vi "UHR-Fleezers Control (host) -Leonardo 04-2018 V3.vi"(0 "Tab Control":T5(tab)=enum."Trap Control (RF)") -> ()   [LabVIEW 2013] (continued)
  n81 = local write "Update Count (MCL)"(w134) -> ()
  n82 = local write "Total Counts (ticks)"(w134) -> ()
  n83 = local write "Ave. Period (s)"(w200) -> ()
  n84 = property on="2D or 1D Scan" class="Bool (strict)"("Val(Sgnl)"=w154) -> ()  [unwired: 2 in, 2 out]
  n85 = xnode "Read/Write Control"("FPGA VI Reference In"=w151, "error in"=w171, "ai count"="AI Count (ticks)", "Interlace ON/OFF"=w137, "Number Interlace Cycles"=w136, "Set 1"=w14, "Set 2"=w13, "Set 3"=w12, "FB On/Off Set 1"=w258, "FB On/Off Set 2"=w257, "Interlace Off Parameters"=w135, "FB Setpoint Set 1"=w249, "FB Setpoint Set 2"=w248, "FB Gains"="PID gains", "FB output range"=cluster{"output high":i16, "output low":i16} {"output high"=3000, "output low"=0} ("FB output range 1"), "Cycles per step"=w234, "Scan BD"=w246, "Number of scans"=w230, "Scan steps"=w235, "Scan freq.  increment"=w236, "AO1 (Y)"=w218, "AO2 (X)"=w217, "Scan freq.  increment (MCL)"=w211, "Scan steps (MCL)"=w210, "Cycles per step (MCL)"=w209, "Number of scans (MCL)"=w208, "MCL count"=w134, "Cont. Scan (MCL)"=w207, "MCL Scan Axis"=w201, "1D or 2D Scan?"=w154, "N of AI1 Int Acq Sets"=w191, "BD 1 Delay (ticks)"="Freq switch delay", "Amp switch delay"="Amp switch delay", "Swap F1 and F2"="Swap F1 and F2", "APD Acq Rate Count"=w159, "APD to FIFO"=FALSE, "APD Gate Operating Mode"="APD Gate", "APD Gate ON Count"="APD Gate ON Count", "APD Gate OFF Count"="APD Gate OFF Count", "Invert APD Gate"="Invert APD Gate", "DIO count 1 (ticks)"="DIO count 1 (ticks)", "DIO count 2 (ticks)"="DIO count 2 (ticks)", "DIO count 3 (ticks)"="DIO count 3 (ticks)", "APD 1 AO scale factor"="APD 1 AO Mult.", "APD 2 AO scale factor"="APD 2 AO Mult.", "Diff FB Measurement?"=w19, "Dynamic Force FB (Ronen)"=w18, "Negate Diff?"=w17, "Next trap write delay (ticks)"="Next trap write delay (ticks)", "Phase offset method"="Phase offset method", "Phase Trap 1"="Phase increment trap 1", "RF phase reset before cycles"="RF phase reset before cycles", "Phase Trap 2"="Phase increment trap 2") -> ("FPGA VI Reference Out"=w129:T20, "error out"=w131:errorcluster)  [unwired: 1 in]
  n86 = local read "Green Laser ON/Interlacing"() -> (w132:bool)
  n87 = local read "Green laser mode"() -> (w133:enum32{"Laser ON", "Laser OFF", "Interlace"})
  n88 = local read "GI Frequency, OFF count"() -> (w125:u32)
  n89 = local read "GI Frequency, ON count"() -> (w124:u32)
  n90 = Multiply(x="Current When FB OFF (%)", y=655.35) -> (x*y=w115:dbl)
  n91 = local read "Green FB Count"() -> (w123:u32)
  n92 = Multiply(x="Green FB Setpoint (mV)", y=3.2767) -> (x*y=w112:dbl)
  n93 = To Unsigned Word Integer(number=w115) -> (unsigned 16bit integer=w113:u16)
  n94 = local read "Invert GI"() -> (w127:bool)
  n95 = To Word Integer(number=w112) -> (16bit integer=w110:i16)
  n96 = case shown="True" w132 {
    tunnel: w133 -> [_ w293]
    tunnel: [enum32{"Laser ON", "Laser OFF", "Interlace"}."Laser OFF" ("Green laser mode") w293] -> w126
    frame False {
    }
    frame True {
    }
  }
  n97 = local read "Trap Pos. AI1 X Pre-scale"() -> (w81:u16)
  n98 = local read "Trap Pos FB Monitor\nT1 or T2"() -> (w88:bool)
  n99 = local read "Trap Pos FB Int Count"() -> (w76:u16)
  n100 = local read "Trap Pos FB Negate Action"() -> (w87:bool)
  n101 = local read "Trap Pos. FB Offset Factor"() -> (w86:i64)
  n102 = local read "Trap Pos. FB Mult Factor"() -> (w85:i64)
  n103 = local read "Trap Pos. FB Gains"() -> (w83:T11)
  n104 = local read "Trap Pos. FB Range"() -> (w84:T12)
  n105 = xnode "Read/Write Control"("FPGA VI Reference In"=w129, "error in"=w131, "Green interlace ON count 2"=w124, "Green interlace OFF count 2"=w125, "Invert GI 2"=w127, "Operating Mode 2"=w126, "Green FB Gains"="Green FB Gains", "Green FB Setpoint"=w110, "Green FB On/Off"="Green FB On/Off", "Current Out"=w113, "Green int current ON count adj"="Green int current ON count adj", "Green FB Count"=w123, "Operating Mode"=w126, "Green interlace OFF count"=w125, "Green interlace ON count"=w124, "Invert GI"=w127, "Trap Pos FB Monitor T1 or T2"=w88, "Trap Pos FB Negate Action"=w87, "Trap Pos. FB Offset Factor"=w86, "Trap Pos. FB Mult Factor"=w85, "Trap pos. FB Range"=w84, "Trap Pos. FB Gains"=w83, "Force feedback"=FALSE, "AI1 X Scale"=w81, "Trap Pos to FIFO"=TRUE, "Trap Pos FB Int Count"=w76) -> ("FPGA VI Reference Out"=w128:T20, "error out"=w130:errorcluster)
  n106 = xnode "Invoke Method"("FPGA VI Reference In"=w128, "error in"=w130, "Requested Depth"="Trap AI FIFO Depth") -> ("FPGA VI Reference Out"=w91:T20, "error out"=w90:errorcluster)  [unwired: 1 out]
  n107 = xnode "Invoke Method"("FPGA VI Reference In"=w91, "error in"=w90, "Requested Depth"="Trap Position FIFO Depth") -> ("FPGA VI Reference Out"=w78:T20, "error out"=w77:errorcluster)  [unwired: 1 out]
  n108 = flat-sequence {
    tunnel: w152 -> [w298]
    tunnel: [w298] -> w151
    tunnel: [w297] -> w35
    tunnel: [w296] -> w150
    tunnel: [w294] -> w148
    tunnel: [w295] -> w149
    frame #0 {
      w295 = T16 {"Minimum"=60.0, "Maximum"=90.0, "Increment"=1.0} ("Min Max Inc")
      w294 = T16 {"Minimum"=0.0, "Maximum"=75.0, "Increment"=1.0} ("Data Entry Limits")
      w297 = T16 {"Minimum"=60.0, "Maximum"=90.0, "Increment"=1.0} ("Min Max Inc")
      w296 = T16 {"Minimum"=0.0, "Maximum"=75.0, "Increment"=1.0} ("Data Entry Limits")
      n109 = property on="BD 2 Frequency 1 (MHz)" class="DigNum (strict)"("Data Range"=w295) -> ()  [unwired: 2 in, 2 out]
      n110 = property on="BD 2 Frequency 3 (MHz)" class="DigNum (strict)"("Data Range"=w295) -> ()  [unwired: 2 in, 2 out]
      n111 = property on="BD 2 Frequency 2 (MHz)" class="DigNum (strict)"("Data Range"=w295) -> ()  [unwired: 2 in, 2 out]
      n112 = property on="BD 1 Frequency 1 (MHz)" class="DigNum (strict)"("Data Range"=w297) -> ()  [unwired: 2 in, 2 out]
      n113 = property on="BD 1 Frequency 2 (MHz)" class="DigNum (strict)"("Data Range"=w297) -> ()  [unwired: 2 in, 2 out]
      n114 = property on="BD 1 Frequency 3 (MHz)" class="DigNum (strict)"("Data Range"=w297) -> ()  [unwired: 2 in, 2 out]
      n115 = property on="BD 2 Amplitude 1 (%)" class="DigNum (strict)"("Data Range"=w294) -> ()  [unwired: 2 in, 2 out]
      n116 = property on="BD 2 Amplitude 2 (%)" class="DigNum (strict)"("Data Range"=w294) -> ()  [unwired: 2 in, 2 out]
      n117 = property on="BD 2 Amplitude 3 (%)" class="DigNum (strict)"("Data Range"=w294) -> ()  [unwired: 2 in, 2 out]
      n118 = property on="BD 1 Amplitude 3 (%)" class="DigNum (strict)"("Data Range"=w296) -> ()  [unwired: 2 in, 2 out]
      n119 = property on="BD 1 Amplitude 2 (%)" class="DigNum (strict)"("Data Range"=w296) -> ()  [unwired: 2 in, 2 out]
      n120 = property on="BD 1 Amplitude 1 (%)" class="DigNum (strict)"("Data Range"=w296) -> ()  [unwired: 2 in, 2 out]
      "X RF Frequency Limits (MHz)" <- w297
      "X RF Amplitude Limits (%)" <- w296
      "Y RF Amplitude Limits (%)" <- w294
      "Y RF Frequency Limits (MHz)" <- w295
    }
  }
  n121 = xnode "Invoke Method"("FPGA VI Reference In"=w78, "error in"=w77) -> ("FPGA VI Reference Out"=w55:T20, "error out"=w54:errorcluster)  [unwired: 1 in]
  n122 = flat-sequence "Initial FPGA Loop Relative Phase Adjustment" {
    tunnel: "Initial Phase Adjustment (APD 2 Gate)" -> [w300]
    tunnel: "Initial Phase Adjustment (GI) 2" -> [w301]
    tunnel: "Initial Phase Adj. (MCL)" -> [w302]
    tunnel: w54 -> [w303]
    tunnel: w55 -> [w304]
    tunnel: "Initial Phase Adjustment (GI)" -> [w305]
    tunnel: "Initial Phase Adjustment (AI1)" -> [w306]
    tunnel: [w306] -> w64
    tunnel: [w305] -> w63
    tunnel: [w304] -> w62
    tunnel: [w303] -> w61
    tunnel: [w302] -> w60
    tunnel: [w301] -> w59
    tunnel: [w300] -> w58
    tunnel: [w318] -> w177
    tunnel: [w312] -> w175
    tunnel: "Initial Phase Adjustment (APD Acq)" -> [w311]
    tunnel: "Initial Phase Adjustment (APD 1 Gate)" -> [w310]
    tunnel: "Initial Phase Adjustment (Green FB)" -> [w309]
    tunnel: w64 -> [w317]
    tunnel: w63 -> [w316]
    tunnel: w62 -> [w315]
    tunnel: w61 -> [w314]
    tunnel: w60 -> [w313]
    tunnel: w59 -> [w308]
    tunnel: w58 -> [w307]
    tunnel: w177 -> [w320]
    tunnel: [w321] -> w176
    tunnel: w175 -> [w321]
    tunnel: [w320] -> w174
    tunnel: w176 -> [w324]
    tunnel: w174 -> [w323]
    tunnel: [w326] -> w173
    tunnel: [w325] -> w172
    tunnel: [w328] -> w53
    tunnel: [w329] -> w56
    tunnel: w173 -> [w329]
    tunnel: w172 -> [w328]
    frame #0 {
      n123 = Wait (ms)(milliseconds to wait=u32 1000) -> ()  [unwired: 1 out]
    }
    frame #1 {
      n124 = xnode "Read/Write Control"("FPGA VI Reference In"=w315, "error in"=w314, "Phase count adjustment"=w317, "Phase count adjustment (GI)"=w316, "Phase count adjustment (MCL)"=w313, "Phase Count Adjustment (APD Acq)"=w311, "Phase count adjustment (APD 1 Gate)"=w310, "Phase count adjustment (APD 2 Gate)"=w307, "Phase count adjustment (Green FB)"=w309, "Phase count adjustment (GI) 2"=w308) -> ("FPGA VI Reference Out"=w312:T20, "error out"=w318:errorcluster)
    }
    frame #2 {
      n125 = Wait (ms)(milliseconds to wait=u32 1000) -> ()  [unwired: 1 out]
    }
    frame #3 {
      w322 = TRUE
      n126 = xnode "Read/Write Control"("FPGA VI Reference In"=w324, "error in"=w323, "+ phase"=w322, "+ phase (GI)"=w322, "+ phase (MCL)"=w322, "+ phase (APD Acq)"=w322, "+ phase (APD 1 Gate)"=w322, "+ phase (APD 2 Gate)"=w322, "+ phase (Green FB)"=w322, "+ phase (GI) 2"=w322) -> ("FPGA VI Reference Out"=w325:T20, "error out"=w326:errorcluster)
    }
    frame #4 {
      n127 = Wait (ms)(milliseconds to wait=u32 1000) -> ()  [unwired: 1 out]
    }
  }
  n128 = Unbundle By Name(w35) -> ("Minimum"=w34:dbl, "Maximum"=w33:dbl)
  n129 = local read "Phase adj. (Green FB)"() -> (w146:i16)
  n130 = local read "Phase adj. (GI) 2"() -> (w116:i16)
  n131 = local read "Phase adjust (MCL)"() -> (w202:i16)
  n132 = local read "Phase adj. (AI1)"() -> (w204:i16)
  n133 = local read "Phase adj. (GI)"() -> (w203:i16)
  n134 = Multiply(x=w34, y=w32) -> (x*y=w30:dbl)
  n135 = Multiply(x=w33, y=w32) -> (x*y=w31:dbl)
  n136 = Multiply(x=49152000.0, y=6.0) -> (x*y=w24:dbl)
  n137 = Scale By Power Of 2(n=w29, x=w30) -> (x*2^n=w26:dbl)
  n138 = Scale By Power Of 2(n=w29, x=w31) -> (x*2^n=w25:dbl)
  n139 = xnode "Read/Write Control"("FPGA VI Reference In"=w53, "error in"=w56, "Phase count adjustment"=w204, "Phase count adjustment (GI)"=w203, "Phase count adjustment (MCL)"=w202, "Phase Count Adjustment (APD Acq)"="Phase Adj. (APD Acq)", "Phase count adjustment (APD 1 Gate)"="Phase Adj. (APD 1 Gate)", "Phase count adjustment (APD 2 Gate)"="Phase Adj. (APD 2 Gate)", "Phase count adjustment (Green FB)"=w146, "Phase count adjustment (GI) 2"=w116) -> ("FPGA VI Reference Out"=w4:T20, "error out"=w10:errorcluster)
  n140 = Divide(x=w25, y=w24) -> (x/y=w22:dbl)
  n141 = Divide(x=w26, y=w24) -> (x/y=w23:dbl)
  n142 = To Unsigned Quad Integer(1:w23) -> (0:w21:u64)
  n143 = To Unsigned Quad Integer(1:w22) -> (0:w20:u64)
  n144 = xnode "Read/Write Control"("FPGA VI Reference In"=w4, "FB Min frequency"=w21, "FB Max Frequency"=w20) -> ()  [unwired: 1 in, 2 out]
  n145 = call "set RF board frequency - interlace.vi"("Board 2 Frequency Limits"=w149, "Board 1 Frequency Limits"=w35, "error in"=w10, "FPGA VI Reference In"=w4, "Board 2 Frequency 3 (MHz)"="BD 2 Frequency 3 (MHz)", "Board 1 Frequency 3 (MHz)"="BD 1 Frequency 3 (MHz)", "Board 2 Frequency 2 (MHz)"="BD 2 Frequency 2 (MHz)", "Board 2 Frequency 1 (MHz)"="BD 2 Frequency 1 (MHz)", "Board 1 Frequency 2 (MHz)"="BD 1 Frequency 2 (MHz)", "Board 1 Frequency 1  (MHz)"="BD 1 Frequency 1 (MHz)") -> ("error out"=w269:errorcluster, "FPGA VI Reference Out"=w270:T20)
  n146 = xnode "Read/Write Control"("FPGA VI Reference In"=w4, "Number of ON cycles"="Cycles ON", "Number of OFF cycles"="Cycles OFF", "Green long-scale interlacing"="Long - scale interlacing") -> ()  [unwired: 1 in, 2 out]
  n147 = call "set RF board amplitude - interlace.vi"("Board 2 Amplitude Limits"=w148, "Board 1 Amplitude Limits"=w150, "error in"=w269, "FPGA VI Reference In"=w270, "Board 2 Amplitude 3 (%)"="BD 2 Amplitude 3 (%)", "Board 1 Amplitude 3 (%)"="BD 1 Amplitude 3 (%)", "Board 2 Amplitude 2 (%)"="BD 2 Amplitude 2 (%)", "Board 2 Amplitude 1 (%)"="BD 2 Amplitude 1 (%)", "Board 1 Amplitude 2 (%)"="BD 1 Amplitude 2 (%)", "Board 1 Amplitude 1 (%)"="BD 1 Amplitude 1 (%)") -> ("error out"=w51:errorcluster, "FPGA VI Reference Out"=w52:T20)
  n148 = flat-sequence {
    tunnel: w52 -> [w331]
    tunnel: w51 -> [w330]
    tunnel: [w331] -> w262
    tunnel: [w330] -> w261
    tunnel: [w339] -> w260
    tunnel: w262 -> [w339]
    tunnel: [w338] -> w259
    tunnel: w261 -> [w338]
    tunnel: w260 -> [w342]
    tunnel: w259 -> [w341]
    tunnel: [w342] -> w47
    tunnel: [w341] -> w46
    tunnel: [w348] -> w73
    tunnel: [w352] -> w57
    tunnel: w47 -> [w352]
    tunnel: w46 -> [w347]
    frame #0 {
      n149 = local read "Trap 1 (ON/OFF)"() -> (w332:bool)
      n150 = local write "Saving..."(FALSE ("Saving Data")) -> ()
      n151 = local write "Stop All"(FALSE ("Stop All")) -> ()
      n152 = local write "Index"(1.0 ("Index")) -> ()
      n153 = property on="Trap 1 ON" class="Bool (strict)"("Value"=w332) -> ()  [unwired: 2 in, 2 out]
      "Manipulating Trap" <- FALSE ("Manipulating Trap")
    }
    frame #1 {
      n154 = local read "Trap 2 (ON/OFF)"() -> (w337:bool)
      n155 = Wait (ms)(milliseconds to wait=u32 50) -> ()  [unwired: 1 out]
      n156 = property on="Trap 2 ON" class="Bool (strict)"("Val(Sgnl)"=w337) -> ()  [unwired: 2 in, 2 out]
    }
    frame #2 {
      n157 = local read "Scan Range (nm)"() -> (w343:dbl)
      n158 = call "Update messages.vi"("Message to add"="UHR-Fleezers ready.", "Old message string"="") -> ("New message string"=w346:string)
      n159 = local write "Messages"(w346) -> ()
      n160 = property on="Scan Range (nm)" class="DigNum (strict)"("Val(Sgnl)"=w343) -> ()  [unwired: 2 in, 2 out]
    }
    frame #3 {
      n161 = call "hamilton_controller.vi"("error in"=w347, "action"=T21."CONNECT") -> ("error out"=w349:errorcluster)  [unwired: 9 in]
      n162 = call "hamilton_controller.vi"("error in"=w349, "action"=T21."INITIALIZE VALVES") -> ("error out"=w348:errorcluster)  [unwired: 9 in]
    }
  }
  n163 = Subtract(x="BD 1 Frequency 1 (MHz)", y="BD 1 Frequency 2 (MHz)") -> (x-y=w190:dbl)
  n164 = Subtract(x="BD 2 Frequency 1 (MHz)", y="BD 2 Frequency 2 (MHz)") -> (x-y=w189:dbl)
  n165 = Square(x=w189) -> (x^2=w187:dbl)
  n166 = Square(x=w190) -> (x^2=w188:dbl)
  n167 = Add(x=w188, y=w187) -> (x+y=w186:dbl)
  n168 = Square Root(x=w186) -> (sqrt(x)=w185:dbl)
  n169 = local write "Trap Delta (MHz)"(w185) -> ()
  n170 = call "IMAQ Create"("Image Name"="APD 1 Image", "Image Type"=w97) -> ("New Image"=w96:T3)  [unwired: 3 in, 1 out]
  n171 = call "IMAQ Create"("Image Name"="APD 2 Image", "Image Type"=w97) -> ("New Image"=w95:T3)  [unwired: 3 in, 1 out]
  n172 = call "IMAQ Create"("Image Name"="Det. X Image", "Image Type"=w97) -> ("New Image"=w94:T3)  [unwired: 3 in, 1 out]
  n173 = call "IMAQ Create"("Image Name"="Det. Y Image", "Image Type"=w97) -> ("New Image"=w93:T3)  [unwired: 3 in, 1 out]
  n174 = Bundle("New Image"=w96, "New Image"=w95, "New Image"=w94, "New Image"=w93) -> (w92:T22)  [unwired: 1 in]
  n175 = Current VI's Path() -> (path=w36:path)
  n176 = Concatenate Strings("N.D.", "\r\n") -> (w40:string)
  n177 = Strip Path(path=w36) -> (stripped path=w37:path)  [unwired: 1 out]
  n178 = Initialize Array(w40, 4, 3) -> (w43:string[][])
  n179 = Build Path(base path=w37, name or relative path="Locations.txt") -> (appended path=→"Location path":path)
  n180 = local write "Location Matrix"(w43) -> ()
  n181 = while {
    stop <- w353 stop-if-true
    n182 = event shown="[0] Timeout" {
      selector: _ -> [_ _ _ _ _ _ _ _]
      dyn-events: _ -> [_ _ _ _ _ _ _ _]
      timeout: 10 -> [_ _ _ _ _ _ _ _]
      tunnel: [FALSE _ _ _ _ _ _ TRUE] -> w353
      event Timeout {
        # "Change the trajectory mode to Jog"
        # "Query and display stage positions"
        # "Setting ESP300 left and right limits for Z-axis, input in mm"
        # "Display Selected Location"
        n183 = event-data() -> ()  [unwired: 1 in, 2 out]
        n184 = local read "Capture Locations"() -> (w378:i32)
        n185 = local read "Location Matrix"() -> (w379:string[][])
        n186 = Concatenate Strings("1TP;\n2TP;\n3TP;\n1MD?;\n2MD?;\n3MD?" ("Substring"), "\r") -> (w362:string)
        n187 = local read "ESP Port"() -> (w365:refnum<visa-resource-name>)
        n188 = Index Array(array=w379, index (row)=w378) -> (element=w377:string[])  [unwired: 1 in]
        n189 = local read "ESP Port"() -> (w374:refnum<visa-resource-name>)
        n190 = VISA Write(VISA resource name=w365, write buffer=w362, error in (no error)="error in") -> (VISA resource name out=w363:refnum<visa-resource-name>, error out=w361:errorcluster)  [unwired: 1 out]
        n191 = Concatenate Strings("3SL" ("Substring"), "ESP ZL-Limit", ";3SR", "ESP ZR-Limit", "\r") -> (w373:string)
        n192 = Array To Cluster(array=w377) -> (cluster=w376:T23)
        n193 = case shown="True" TRUE ("Case Constant\n(See Context Help)") {
          tunnel: w363 -> [_ w417]
          tunnel: w361 -> [w398 w416]
          tunnel: [w398 w400] -> w367
          frame False {
          }
          frame True {
            w410 = u16 10 items=["1.0"=10, "1.5"=15, "2.0"=20] ("Serial Settings:Stop Bits")
            w411 = u16 0 items=["None", "Odd", "Even", "Mark", "Space"] ("Serial Settings:Parity")
            n194 = property class="Instr"(reference=w417, error in=w416, "Baud"=u32 921600 ("Serial Settings:Baud Rate"), "Data Bits"=u16 8 ("Serial Settings:Data Bits"), "Parity"=w411, "Stop Bits"=w410) -> (reference out=w415:refnum<visa-resource-name>, error out=w414:errorcluster, "Bytes at Port"=w399:u32)
            n195 = Wait (ms)(milliseconds to wait=u32 10) -> ()  [unwired: 1 out]
            n196 = VISA Read(VISA resource name=w415, byte count=w399, error in (no error)=w414) -> (VISA resource name out=w423:refnum<visa-resource-name>, read buffer=→"X Pos":string, error out=w424:errorcluster)  [unwired: 1 out]
            n197 = VISA Read(VISA resource name=w423, byte count=w399, error in (no error)=w424) -> (VISA resource name out=w421:refnum<visa-resource-name>, read buffer=→"Y Pos":string, error out=w422:errorcluster)  [unwired: 1 out]
            n198 = VISA Read(VISA resource name=w421, byte count=w399, error in (no error)=w422) -> (VISA resource name out=w409:refnum<visa-resource-name>, read buffer=→"Z Pos Pos":string, error out=w408:errorcluster)  [unwired: 1 out]
            n199 = VISA Read(VISA resource name=w409, byte count=w399, error in (no error)=w408) -> (VISA resource name out=w405:refnum<visa-resource-name>, read buffer=→"X Motion":string, error out=w406:errorcluster)  [unwired: 1 out]
            n200 = VISA Read(VISA resource name=w405, byte count=w399, error in (no error)=w406) -> (VISA resource name out=w404:refnum<visa-resource-name>, read buffer=→"Y Motion":string, error out=w402:errorcluster)  [unwired: 1 out]
            n201 = VISA Read(VISA resource name=w404, byte count=w399, error in (no error)=w402) -> (read buffer=→"Z motion":string, error out=w400:errorcluster)  [unwired: 2 out]
          }
        }
        "error out" <- w367
        n202 = VISA Write(VISA resource name=w374, write buffer=w373) -> ()  [unwired: 1 in, 3 out]
        n203 = local write item#483(w376) -> ()
        n204 = disable-structure shown="Disabled" {
          frame Disabled {
            # "Change Low Jog Velocity"
            # "Change High Jog Velocity"
            n205 = Concatenate Strings("1JH" ("Substring"), "Axis 1", "2JH" ("Substring"), "Axis 2", "3JH" ("Substring"), "Axis 3", "\r") -> (w397:string)
            n206 = local read "ESP Port"() -> (w396:refnum<visa-resource-name>)
            n207 = VISA Write(VISA resource name=w396, write buffer=w397) -> ()  [unwired: 1 in, 3 out]
            n208 = Concatenate Strings("1JW" ("Substring"), "Axis 1", "2JW" ("Substring"), "Axis 2", "3JW" ("Substring"), "Axis 3", "\r") -> (w388:string)
            n209 = local read "ESP Port"() -> (w387:refnum<visa-resource-name>)
            n210 = VISA Write(VISA resource name=w387, write buffer=w388) -> ()  [unwired: 1 in, 3 out]
          }
          frame Enabled {
          }
        }
        n211 = local read "ESP Port"() -> (w355:refnum<visa-resource-name>)
        n212 = Concatenate Strings("1TJ3;\n2TJ3;\n3TJ3" ("Substring"), "\r") -> (w356:string)
        n213 = VISA Write(VISA resource name=w355, write buffer=w356) -> ()  [unwired: 1 in, 3 out]
      }
      event "Goto Top (F6)": Value Change {
        n214 = event-data() -> ()  [unwired: 1 in, 5 out]
        n215 = stacked-sequence {
          frame #0 {
            # "stop motions of all axes before going to avoid reversing of direction"
            n216 = local read "ESP Port"() -> (w429:refnum<visa-resource-name>)
            n217 = Concatenate Strings("ST" ("Substring"), "\r") -> (w426:string)
            n218 = VISA Write(VISA resource name=w429, write buffer=w426) -> ()  [unwired: 1 in, 3 out]
          }
          frame #1 {
            n219 = Wait (ms)(milliseconds to wait=u32 50) -> ()  [unwired: 1 out]
          }
          frame #2 {
            # "Change the trajectory mode to Trapezoidal"
            n220 = local read "ESP Port"() -> (w434:refnum<visa-resource-name>)
            n221 = Concatenate Strings("1TJ1;\n2TJ1;\n3TJ1" ("Substring"), "\r") -> (w431:string)
            n222 = VISA Write(VISA resource name=w434, write buffer=w431) -> ()  [unwired: 1 in, 3 out]
          }
          frame #3 {
            # "Go to Top Dispensor"
            n223 = local read "Location Matrix"() -> (w446:string[][])
            n224 = Index Array(array=w446, index (row)=0) -> (element=w442:string[])  [unwired: 1 in]
            n225 = Decimate 1D Array(w442) -> (w440:string[], w438:string[], w436:string[])
            n226 = local read "ESP Port"() -> (w443:refnum<visa-resource-name>)
            n227 = Concatenate Strings("1PA" ("Substring"), w440, "2PA" ("Substring"), w438, "3PA" ("Substring"), w436, "\r") -> (w444:string)
            n228 = VISA Write(VISA resource name=w443, write buffer=w444) -> ()  [unwired: 1 in, 3 out]
          }
          frame #4 {
            n229 = Wait (ms)(milliseconds to wait=u32 100) -> ()  [unwired: 1 out]
          }
          frame #5 {
            # "Change the trajectory mode to Jog"
            n230 = local read "ESP Port"() -> (w451:refnum<visa-resource-name>)
            n231 = Concatenate Strings("1TJ3;\n2TJ3;\n3TJ3" ("Substring"), "\r") -> (w448:string)
            n232 = VISA Write(VISA resource name=w451, write buffer=w448) -> ()  [unwired: 1 in, 3 out]
          }
        }
      }
      event "Goto Exp (F8)": Value Change {
        n233 = event-data() -> ()  [unwired: 1 in, 5 out]
        n234 = stacked-sequence {
          frame #0 {
            # "stop motions of all axes before going to avoid reversing of direction"
            n235 = local read "ESP Port"() -> (w455:refnum<visa-resource-name>)
            n236 = Concatenate Strings("ST" ("Substring"), "\r") -> (w452:string)
            n237 = VISA Write(VISA resource name=w455, write buffer=w452) -> ()  [unwired: 1 in, 3 out]
          }
          frame #1 {
            n238 = Wait (ms)(milliseconds to wait=u32 50) -> ()  [unwired: 1 out]
          }
          frame #2 {
            # "Change the trajectory mode to Trapezoidal"
            n239 = local read "ESP Port"() -> (w460:refnum<visa-resource-name>)
            n240 = Concatenate Strings("1TJ1;\n2TJ1;\n3TJ1" ("Substring"), "\r") -> (w457:string)
            n241 = VISA Write(VISA resource name=w460, write buffer=w457) -> ()  [unwired: 1 in, 3 out]
          }
          frame #3 {
            # "Go to Experimental"
            n242 = local read "Location Matrix"() -> (w472:string[][])
            n243 = Index Array(array=w472, index (row)=2) -> (element=w468:string[])  [unwired: 1 in]
            n244 = Decimate 1D Array(w468) -> (w466:string[], w464:string[], w462:string[])
            n245 = Concatenate Strings("1PA" ("Substring"), w466, "2PA" ("Substring"), w464, "3PA" ("Substring"), w462, "\r") -> (w470:string)
            n246 = local read "ESP Port"() -> (w469:refnum<visa-resource-name>)
            n247 = VISA Write(VISA resource name=w469, write buffer=w470) -> ()  [unwired: 1 in, 3 out]
          }
          frame #4 {
            n248 = Wait (ms)(milliseconds to wait=u32 200) -> ()  [unwired: 1 out]
          }
          frame #5 {
            # "Change the trajectory mode to Jog"
            n249 = local read "ESP Port"() -> (w474:refnum<visa-resource-name>)
            n250 = Concatenate Strings("1TJ3;\n2TJ3;\n3TJ3" ("Substring"), "\r") -> (w477:string)
            n251 = VISA Write(VISA resource name=w474, write buffer=w477) -> ()  [unwired: 1 in, 3 out]
          }
        }
      }
      event "Goto Bottom (F7)": Value Change {
        n252 = event-data() -> ()  [unwired: 1 in, 5 out]
        n253 = stacked-sequence {
          frame #0 {
            # "stop motions of all axes before going to avoid reversing of direction"
            n254 = local read "ESP Port"() -> (w481:refnum<visa-resource-name>)
            n255 = Concatenate Strings("ST" ("Substring"), "\r") -> (w478:string)
            n256 = VISA Write(VISA resource name=w481, write buffer=w478) -> ()  [unwired: 1 in, 3 out]
          }
          frame #1 {
            n257 = Wait (ms)(milliseconds to wait=u32 50) -> ()  [unwired: 1 out]
          }
          frame #2 {
            # "Change the trajectory mode to Trapezoidal"
            n258 = local read "ESP Port"() -> (w486:refnum<visa-resource-name>)
            n259 = Concatenate Strings("1TJ1;\n2TJ1;\n3TJ1" ("Substring"), "\r") -> (w483:string)
            n260 = VISA Write(VISA resource name=w486, write buffer=w483) -> ()  [unwired: 1 in, 3 out]
          }
          frame #3 {
            # "Go to Bottom Dispensor"
            n261 = local read "Location Matrix"() -> (w498:string[][])
            n262 = Index Array(array=w498, index (row)=1) -> (element=w494:string[])  [unwired: 1 in]
            n263 = Decimate 1D Array(w494) -> (w492:string[], w490:string[], w488:string[])
            n264 = Concatenate Strings("1PA" ("Substring"), w492, "2PA" ("Substring"), w490, "3PA" ("Substring"), w488, "\r") -> (w496:string)
            n265 = local read "ESP Port"() -> (w495:refnum<visa-resource-name>)
            n266 = VISA Write(VISA resource name=w495, write buffer=w496) -> ()  [unwired: 1 in, 3 out]
          }
          frame #4 {
            n267 = Wait (ms)(milliseconds to wait=u32 200) -> ()  [unwired: 1 out]
          }
          frame #5 {
            # "Change the trajectory mode to Jog"
            n268 = local read "ESP Port"() -> (w500:refnum<visa-resource-name>)
            n269 = Concatenate Strings("1TJ3;\n2TJ3;\n3TJ3" ("Substring"), "\r") -> (w503:string)
            n270 = VISA Write(VISA resource name=w500, write buffer=w503) -> ()  [unwired: 1 in, 3 out]
          }
        }
      }
      event "Capture": Value Change {
        n271 = event-data() -> ()  [unwired: 1 in, 5 out]
        n272 = local read "Capture Locations"() -> (w504:i32)
        n273 = local read "Z Pos Pos"() -> (w505:string)
        n274 = local read "X Pos"() -> (w507:string)
        n275 = local read "Y Pos"() -> (w506:string)
        n276 = case shown="1" w504 {
          selector: w504 -> [w511 w518 w525 w532]
          tunnel: w507 -> [w514 w521 w528 w535]
          tunnel: w506 -> [w513 w520 w527 w534]
          tunnel: w505 -> [w512 w519 w526 w533]
          frame 0, Default {
            # "Capture Top Dispensor Location"
            n277 = local read "Location Matrix"() -> (w510:string[][])
            n278 = Build Array(w514, w513, w512) -> (w509:string[])
            n279 = Replace Array Subset(array=w510, new element=w509, index (row)=w511) -> (w508:string[][])  [unwired: 1 in]
            n280 = local write "Location Matrix"(w508) -> ()
          }
          frame 1 {
            # "Capture Bottom Dispensor Location"
            n281 = local read "Location Matrix"() -> (w517:string[][])
            n282 = Build Array(w521, w520, w519) -> (w516:string[])
            n283 = Replace Array Subset(array=w517, new element=w516, index (row)=w518) -> (w515:string[][])  [unwired: 1 in]
            n284 = local write "Location Matrix"(w515) -> ()
          }
          frame 2 {
            # "Capture Experimental Region Location"
            n285 = local read "Location Matrix"() -> (w524:string[][])
            n286 = Build Array(w528, w527, w526) -> (w523:string[])
            n287 = Replace Array Subset(array=w524, new element=w523, index (row)=w525) -> (w522:string[][])  [unwired: 1 in]
            n288 = local write "Location Matrix"(w522) -> ()
          }
          frame 3 {
            # "Capture Other Location"
            n289 = local read "Location Matrix"() -> (w531:string[][])
            n290 = Build Array(w535, w534, w533) -> (w530:string[])
            n291 = Replace Array Subset(array=w531, new element=w530, index (row)=w532) -> (w529:string[][])  [unwired: 1 in]
            n292 = local write "Location Matrix"(w529) -> ()
          }
        }
      }
      event "Save": Value Change {
        # "reshape Location Matrix to 1-D array to write"
        n293 = event-data() -> ()  [unwired: 1 in, 5 out]
        n294 = local read "Location Matrix"() -> (w539:string[][])
        n295 = local read "Location path"() -> (w536:path)
        n296 = Reshape Array(w539, 12) -> (w537:string[])
        n297 = Write to Text File(file (use dialog)=w536, text=w537) -> ()  [unwired: 2 in, 3 out]
      }
      event "Activate Joystick": Value Change {
        # "Change the trajectory mode to Jog"
        n298 = event-data() -> ()  [unwired: 1 in, 5 out]
        n299 = disable-structure shown="Disabled" {
          frame Disabled {
            n300 = case shown="True" "Activate Joystick" {
              frame False {
              }
              frame True {
                # "Change the trajectory mode to Jog"
                n301 = local read "ESP Port"() -> (w548:refnum<visa-resource-name>)
                n302 = Concatenate Strings("1TJ3;\n2TJ3;\n3TJ3" ("Substring"), "\r") -> (w545:string)
                n303 = VISA Write(VISA resource name=w548, write buffer=w545) -> ()  [unwired: 1 in, 3 out]
              }
            }
          }
          frame Enabled {
          }
        }
        n304 = local read "ESP Port"() -> (w540:refnum<visa-resource-name>)
        n305 = Concatenate Strings("1TJ3;\n2TJ3;\n3TJ3" ("Substring"), "\r") -> (w543:string)
        n306 = VISA Write(VISA resource name=w540, write buffer=w543) -> ()  [unwired: 1 in, 3 out]
      }
      event "Stop All": Mouse Down {
        n307 = event-data() -> ()  [unwired: 1 in, 5 out]
      }
    }
  }
  n308 = disable-structure shown="Disabled" {
    disable-tunnel: w57 -> [w578 _]
    frame Disabled {
      w573 = T17 0 items=["Grayscale (U8)", "Grayscale (I16)", "Grayscale (SGL)", "Complex (CSG)", "RGB (U32)", "HSL (U32)", "RGB (U64)", "Grayscale (U16)"] ("Image Type")
      n309 = call <vilib>:"IMAQ Init.vi"("Interface Name"="img0") -> ("error out"=w575:errorcluster, "IMAQ Session Out"=w577:refnum<k11>)  [unwired: 9 in]
      n310 = call <vilib>:"IMAQ Grab Setup.vi"("error in (no error)"=w575, "IMAQ Session In"=w577) -> ("error out"=w571:errorcluster, "IMAQ Session Out"=w572:refnum<k11>)  [unwired: 8 in]
      n311 = call "IMAQ Create"("Image Name"="untitled", "Image Type"=w573) -> ("New Image"=w570:T3)  [unwired: 3 in, 1 out]
      n312 = call <vilib>:"Application Directory.vi"() -> ("Application Directory"=w557:path)
      n313 = Build Path(base path=w557, name or relative path="_trap_screen_positions") -> (appended path=w565:path)
      n314 = Open/Create/Replace File(file path (use dialog)=w565, operation (0:open)=T24."open or create", access (0:read/write)=enum16{"read/write", "read-only", "write-only"}."read/write") -> (refnum out=w567:refnum<file>)  [unwired: 3 in, 2 out]
      n315 = local read "Trap Sets"() -> (w559:u32)
      n316 = for "Load trap positions on video screen from file." {
        N: w559 -> [_]
        tunnel: [w585] -> w560
        tunnel: w567 -> [w584]
        tunnel: [w581] -> w556 mode=indexing
        w583 = 4
        n317 = for {
          N: w583 -> [_]
          tunnel: [w589] -> w585
          tunnel: w584 -> [w588]
          tunnel: w583 -> [w587]
          tunnel: [w586] -> w582 mode=indexing
          n318 = Read from Binary File(5:w587, 11:w588) -> (2:w586:i32, 3:w589:refnum<file>)  [unwired: 4 in, 2 out]
        }
        n319 = Array To Cluster(array=w582) -> (cluster=w581:T28)
      }
      n320 = node-c288() -> (w580:T25)  [unwired: 4 in]
      n321 = timed-loop "acquire video and stage position" {
        timing: w580 -> [_]
        timing-out: [_] -> w579
        tunnel: w572 -> [w608]
        tunnel: w571 -> [w607]
        tunnel: w570 -> [w606]
        tunnel: [w605] -> w552
        tunnel: [w602] -> w553
        tunnel: [w603] -> w551
        tunnel: w578 -> [_]
        shift-right: [w599] -> w569
        shift-left: w556 -> [w600]
        tunnel: w559 -> [w597]
        stop <- w604 stop-if-true
        n322 = node-c288() -> ()  [unwired: 1 in, 1 out]
        n323 = event shown="[0] Timeout" {
          selector: _ -> [_ _ _ _]
          dyn-events: _ -> [_ _ _ _]
          timeout: 10 -> [_ _ _ _]
          tunnel: w608 -> [w619 w634 w643 w662]
          tunnel: w607 -> [w618 w636 w641 w664]
          tunnel: w606 -> [w617 w635 w642 w663]
          tunnel: [w616 w634 w643 w662] -> w605
          tunnel: [w609 w638 FALSE FALSE] -> w604
          tunnel: [w613 w636 w641 w664] -> w603
          tunnel: [w612 w635 w642 w663] -> w602
          tunnel: "radius" -> [_ _ w648 _]
          tunnel: w600 -> [w610 w637 w646 _]
          tunnel: [w610 w637 w647 cluster{i32, i32, i32, i32}[] []] -> w599
          tunnel: w597 -> [_ _ w639 _]
          event Timeout {
            n324 = event-data() -> ()  [unwired: 1 in, 2 out]
            n325 = call <vilib>:"IMAQ Grab Acquire.vi"("error in (no error)"=w618, "Image In"=w617, "IMAQ Session In"=w619) -> ("error out"=w614:errorcluster, "Image Out"=w615:T3, "IMAQ Session Out"=w616:refnum<k11>)  [unwired: 5 in, 1 out]
            n326 = case shown="True" "trap\nmarkers?" {
              tunnel: w610 -> [_ w627]
              tunnel: w615 -> [w621 w626]
              tunnel: w614 -> [w620 w625]
              tunnel: [w620 w624] -> w613
              tunnel: [w621 w622] -> w612
              frame False {
              }
              frame True {
                n327 = for {
                  tunnel: w627 -> [w633] mode=indexing
                  shift-right: [w631] -> w622
                  shift-left: w626 -> [w632]
                  tunnel: w625 -> [w630]
                  tunnel: [w629] -> w624
                  tunnel: u32 16711680 ("Color") -> [w628]
                  n328 = call "IMAQ Overlay Oval"("Color"=w628, "error in (no error)"=w630, "Bounding Rectangle"=w633, "Image"=w632) -> ("error out"=w629:errorcluster, "Image Out"=w631:T3)  [unwired: 6 in]
                }
              }
            }
            "Primary Video Display" <- w612
            n329 = Unbundle By Name(w614) -> ("status"=w609:bool)
          }
          event "Stop All": Value Change {
            n330 = event-data() -> ()  [unwired: 1 in, 5 out]
            n331 = local read "Stop All"() -> (w638:bool)
          }
          event "Primary Video Display": Mouse Down {
            n332 = event-data() -> ()  [unwired: 1 in, 7 out]
            n333 = Array Size(array=w646) -> (size(s)=w645:i32)
            n334 = Less?(x=w645, y=w639) -> (x < y?=w644:bool)
            n335 = case shown="True" w644 {
              tunnel: w648 -> [_ w658]
              tunnel: w646 -> [w649 w652]
              tunnel: [w649 w651] -> w647
              frame False {
              }
              frame True {
                n336 = property on="Primary Video Display" class="ImageControl"() -> ("Last Mouse Position"=w650:cluster{"X":i32, "Y":i32})  [unwired: 2 in, 2 out]
                n337 = Unbundle By Name(w650) -> ("X"=w660:i32, "Y"=w659:i32)
                n338 = Add(x=w659, y=w658) -> (x+y=w656:i32)
                n339 = Subtract(x=w659, y=w658) -> (x-y=w654:i32)
                n340 = Add(x=w660, y=w658) -> (x+y=w655:i32)
                n341 = Subtract(x=w660, y=w658) -> (x-y=w657:i32)
                n342 = Bundle(w657, w656, w655, w654) -> (w653:cluster{i32, i32, i32, i32})  [unwired: 1 in]
                n343 = Build Array (concatenate)(w652, w653) -> (w651:T29)
              }
            }
          }
          event "clear markers": Value Change {
            n344 = event-data() -> ()  [unwired: 1 in, 5 out]
          }
        }
        n345 = node-c288() -> ()  [unwired: 1 in, 1 out]
      }
      n346 = node-c288(w579) -> ()  [unwired: 1 out]
      n347 = Set File Position(offset (in bytes) (0)=i64 0, refnum=w560, from (0:start)=enum16{"start", "end", "current"}."start") -> (refnum out=w561:refnum<file>)  [unwired: 1 in, 1 out]
      n348 = for "Write trap positions to file so they can be remembered\nwhen program is removed from memory" {
        tunnel: w569 -> [w593] mode=indexing
        tunnel: [w591] -> w568
        tunnel: w561 -> [w590]
        n349 = Cluster To Array(cluster=w593) -> (array=w592:i32[])
        n350 = for {
          tunnel: w592 -> [w596] mode=indexing
          tunnel: [w595] -> w591
          tunnel: w590 -> [w594]
          n351 = Write to Binary File(file (use dialog)=w594, data=w596) -> (refnum out=w595:refnum<file>)  [unwired: 4 in, 2 out]
        }
      }
      n352 = Close File(refnum=w568) -> ()  [unwired: 1 in, 2 out]
      n353 = call "IMAQ Dispose"("Image"=w553, "error in (no error)"=w551) -> ("error out"=w550:errorcluster)  [unwired: 4 in]
      n354 = call <vilib>:"IMAQ Stop.vi"("error in (no error)"=w550, "IMAQ Session In"=w552) -> ("error out"=w554:errorcluster, "IMAQ Session Out"=w555:refnum<k11>)  [unwired: 8 in]
      n355 = call <vilib>:"IMAQ Close.vi"("error in (no error)"=w554, "IMAQ Session In"=w555) -> ()  [unwired: 9 in, 1 out]
    }
    frame Enabled {
    }
  }
  n356 = disable-structure shown="Enabled" {
    disable-tunnel: [w671 _] -> w68
    disable-tunnel: w57 -> [w670 _]
    frame Enabled {
      n357 = node-c288() -> (w673:T25)  [unwired: 4 out]
      n358 = timed-loop "Rough control of MCL mirror stage (debugging)" {
        tunnel: w670 -> [w676]
        tunnel: [w675] -> w671
        timing: w673 -> [_]
        timing-out: [_] -> w672
        stop <- w675 stop-if-true
        n359 = node-c288() -> ()  [unwired: 2 out]
        n360 = case shown="0, Default" "MCL Mode" {
          tunnel: w676 -> [_ w679 w726]
          frame 0, Default {
            # "manual positioning"
          }
          frame 1 {
            # "sinusoidal wave"
            n361 = node-c288() -> (w681:T25)  [unwired: 4 out]
            n362 = timed-loop "Oscillate MCL mirror" {
              timing: w681 -> [_]
              timing-out: [_] -> w680
              tunnel: w679 -> [w720]
              i -> [w719]
              stop <- w682 stop-if-true
              n363 = node-c288() -> (w718:i64)  [unwired: 1 out]
              n364 = Multiply(x="AO1", y=32767.0) -> (x*y=w714:dbl)
              n365 = Multiply(x="AO2", y=32767.0) -> (x*y=w709:dbl)
              n366 = Divide(x=w714, y=10.0) -> (x/y=w715:dbl)
              n367 = Divide(x=w709, y=10.0) -> (x/y=w710:dbl)
              n368 = To Word Integer(number=w715) -> (16bit integer=w707:i16)
              n369 = To Word Integer(number=w710) -> (16bit integer=w706:i16)
              n370 = Divide(x=w718, y=i64 1000) -> (x/y=w689:dbl)
              n371 = Multiply(x=w689, y=w719) -> (x*y=w700:dbl)
              n372 = Multiply(x="Osc. freq. (Hz) 2", y=6.283185307179586) -> (x*y=w701:dbl)
              n373 = Multiply(x=w701, y=w700) -> (x*y=w699:dbl)
              n374 = Sine(x=w699) -> (sin(x)=w698:dbl)
              n375 = Multiply(x=w698, y="Osc. amp. (V)") -> (x*y=w696:dbl)
              n376 = Add(x=w696, y="Osc. center (V)") -> (x+y=w694:dbl)
              n377 = Divide(x=w694, y=10.0) -> (x/y=w692:dbl)
              n378 = Multiply(x=w692, y=32767.0) -> (x*y=w687:dbl)
              n379 = Select(t=w687, s="Scan axis", f=w707) -> (s? t:f=w705:dbl)
              n380 = Select(t=w706, s="Scan axis", f=w687) -> (s? t:f=w704:dbl)
              n381 = local read "MCL Mode"() -> (w686:u16)
              n382 = Not Equal?(x=w686, y=u16 1) -> (x != y?=w683:bool)
              n383 = local read "Stop All"() -> (w684:bool)
              n384 = xnode "Read/Write Control"("FPGA VI Reference In"=w720, "AO1 (Y)"=w705, "AO2 (X)"=w704) -> ()  [unwired: 1 in, 2 out]
              n385 = Compound Arithmetic op=OR(w684, w683) -> (w682:bool)
              n386 = node-c288() -> ()  [unwired: 2 out]
            }
            n387 = node-c288(w680) -> ()  [unwired: 1 out]
          }
          frame 2 {
            # "linear scan"
            n388 = case shown="True" "Start Scan" {
              tunnel: w726 -> [_ w738]
              frame False {
              }
              frame True {
                n389 = Subtract(x="End (V)", y="Begin (V)") -> (x-y=w734:dbl)
                n390 = Decrement(x="N Points") -> (x-1=w733:dbl)
                n391 = Divide(x=w734, y=w733) -> (x/y=w731:dbl)
                n392 = for {
                  N: "N Points" -> [_]
                  tunnel: "Begin (V)" -> [w751]
                  tunnel: w738 -> [w743]
                  tunnel: [w742] -> w737 mode=indexing
                  tunnel: w731 -> [w741]
                  tunnel: [w739] -> w730 mode=indexing
                  i -> [w750]
                  n393 = Multiply(x=w741, y=w750) -> (x*y=w749:dbl)
                  n394 = Add(x=w751, y=w749) -> (x+y=w746:dbl)
                  n395 = local read "Scan axis"() -> (w740:bool)
                  n396 = local read "AO1"() -> (w748:dbl)
                  n397 = local read "AO2"() -> (w747:dbl)
                  n398 = Select(t=w746, s=w740, f=w748) -> (s? t:f=w745:dbl)
                  n399 = Select(t=w747, s=w740, f=w746) -> (s? t:f=w744:dbl)
                  n400 = flat-sequence {
                    tunnel: w745 -> [w755]
                    tunnel: w744 -> [w754]
                    tunnel: w743 -> [w752]
                    tunnel: [w765] -> w742
                    tunnel: [w764] -> w739
                    frame #0 {
                      w758 = 10.0 ("y")
                      w753 = 32767.0 ("y")
                      n401 = Multiply(x=w755, y=w753) -> (x*y=w761:dbl)
                      n402 = Multiply(x=w754, y=w753) -> (x*y=w759:dbl)
                      n403 = Divide(x=w761, y=w758) -> (x/y=w762:dbl)
                      n404 = Divide(x=w759, y=w758) -> (x/y=w760:dbl)
                      n405 = To Word Integer(number=w762) -> (16bit integer=w756:i16)
                      n406 = To Word Integer(number=w760) -> (16bit integer=w757:i16)
                      n407 = xnode "Read/Write Control"("FPGA VI Reference In"=w752, "AO1 (Y)"=w756, "AO2 (X)"=w757) -> ()  [unwired: 1 in, 2 out]
                    }
                    frame #1 {
                      n408 = Wait (ms)(milliseconds to wait="DAQ Delay (ms)") -> ()  [unwired: 1 out]
                    }
                    frame #2 {
                      n409 = local read "Slow mean"() -> (w765:dbl)
                      n410 = local read "Sigma"() -> (w764:dbl)
                    }
                  }
                }
                n411 = Bundle("Begin (V)"="Begin (V)", w731, w737) -> (→"MCL Scan":cluster{"Begin (V)":dbl, dbl, dbl[]})  [unwired: 1 out]
                n412 = Bundle("Begin (V)"="Begin (V)", w731, w730) -> (→"MCL Scan 2":cluster{"Begin (V)":dbl, dbl, dbl[]})  [unwired: 1 out]
              }
            }
          }
        }
        n413 = local read "Stop All"() -> (w675:bool)
        n414 = node-c288() -> ()  [unwired: 2 out]
      }
      n415 = node-c288(w672) -> ()  [unwired: 1 out]
    }
    frame Disabled {
    }
  }
  n416 = node-c288(2 ("Processor")) -> (w50:T25)  [unwired: 3 in]
  n417 = timed-loop "Control parameters (event loop)" {
    tunnel: w57 -> [w771]
    shift-right: [w770] -> _
    shift-left: errorcluster {"status"=FALSE, "code"=0, "source"=""} ("error out") -> [w769]
    tunnel: [w768] -> w70
    timing: w50 -> [_]
    timing-out: [_] -> w49
    stop <- w768 stop-if-true
    n418 = node-c288() -> ()  [unwired: 1 in, 1 out]
    n419 = event shown="[60] \"Long - scale interlacing\", \"Cycles ON\", \"Cycles OFF\": Value Change" {
      selector: _ -> [_ _ _ _ _ _ _ _ _ _ _ _ _ _ _ _ _ _ _ _ _ _ _ _ _ _ _ _ _ _ _ _ _ _ _ _ _ _ _ _ _ _ _ _ _ _ _ _ _ _ _ _ _ _ _ _ _ _ _ _ _ _]
      dyn-events: _ -> [_ _ _ _ _ _ _ _ _ _ _ _ _ _ _ _ _ _ _ _ _ _ _ _ _ _ _ _ _ _ _ _ _ _ _ _ _ _ _ _ _ _ _ _ _ _ _ _ _ _ _ _ _ _ _ _ _ _ _ _ _ _]
      timeout: _ -> [_ _ _ _ _ _ _ _ _ _ _ _ _ _ _ _ _ _ _ _ _ _ _ _ _ _ _ _ _ _ _ _ _ _ _ _ _ _ _ _ _ _ _ _ _ _ _ _ _ _ _ _ _ _ _ _ _ _ _ _ _ _]
      tunnel: w771 -> [w812 _ _ _ w849 _ w867 w873 _ _ _ _ w950 _ _ w994 w1000 w1004 w1009 w1045 w1063 w1070 w1088 w1099 w1110 w1121 w1132 w1143 w1161 w1167 w1261 _ w1273 w1311 _ w1371 w1375 w1386 w1391 w1415 _ w1423 _ _ _ _ _ w1559 _ w1576 w1591 w1617 w1620 w1621 w1681 _ w1698 w1700 _ _ w1773 _]
      tunnel: [w811 _ _ _ w839 _ _ w872 _ _ w915 _ w930 _ _ w993 w996 w1003 w1006 w1044 w1061 w1069 w1082 w1093 w1104 w1115 w1126 w1137 w1159 w1166 w1259 _ w1271 w1309 _ w1369 w1373 w1376 w1389 w1413 _ w1421 _ _ _ _ _ w1557 _ _ _ _ _ _ _ _ _ _ _ _ _ _] -> w770
      tunnel: w769 -> [w810 _ _ _ w848 _ _ w871 _ _ w915 _ w949 _ _ w992 w995 w1002 w1005 w1043 w1062 w1068 w1087 w1098 w1109 w1120 w1131 w1142 w1160 w1165 w1260 _ w1272 w1310 _ w1370 w1374 w1385 w1390 w1414 _ w1422 _ _ _ _ _ w1558 _ w1575 w1590 w1616 w1619 w1622 w1680 _ w1697 _ _ _ _ _]
      tunnel: [_ _ _ _ _ _ _ _ _ _ w914 _ _ _ _ _ _ _ _ _ _ _ _ _ _ _ _ _ _ _ _ _ _ _ _ _ _ _ _ _ _ _ _ _ _ _ _ _ _ _ _ _ _ _ _ _ _ _ _ _ _ _] -> w768
      tunnel: [_ _ _ _ _ _ _ _ "Round T1 X" _ _ _ _ _ _ _ _ _ _ _ _ _ _ _ _ _ _ _ _ _ _ _ _ _ _ _ _ _ _ _ _ _ _ _ _ _ _ _ _ _ _ _ _ _ _ _ _ _ _ _ _ _] -> _
      tunnel: [_ _ _ "Adjust Scale\nto Mean" _ _ _ _ _ _ _ _ _ _ _ _ _ _ _ _ _ _ _ _ _ _ _ _ _ _ _ _ _ _ _ _ _ _ _ _ _ _ _ _ _ _ _ _ _ _ _ _ _ _ "Set SP to Reading" _ _ _ _ _ _ _] -> _
      tunnel: [_ _ _ _ _ _ _ _ _ "Round T2 X" _ "Delayed Interlace Start" _ _ _ _ _ _ _ _ _ _ _ _ _ _ _ _ _ _ _ _ _ _ _ _ _ _ _ _ _ _ _ _ _ _ _ _ _ _ _ _ _ _ _ _ _ _ _ _ _ _] -> _
      event "AI Count (ticks)", "Sets to FIFO (Traps)", "Save ave N", "FPGA Ave.", "# Samples/channel", "N sets to save": Value Change {
        # "So that if 'Save ave N' is updated, the AOD scanning code updates too."
        n420 = event-data() -> ()  [unwired: 6 out]
        n421 = local read "AI Count (ticks)"() -> (w793:u32)
        n422 = Unbundle By Name("Sets to FIFO (Traps)") -> ("Set 1"=w776:bool, "Set 2"=w775:bool, "Set 3"=w774:bool)
        n423 = Boolean To (0,1)(Boolean="Sets to FIFO (Traps)") -> (0, 1=w802:cluster{"Set 1":i16, "Set 2":i16, "Set 3":i16})
        n424 = xnode "Read/Write Control"("FPGA VI Reference In"=w812, "error in"=w810, "ai count"=w793, "Set 1"=w776, "Set 2"=w775, "Set 3"=w774, "N of AI1 Int Acq Sets"="N Acq Sets (Traps + Fl.)") -> ("error out"=w811:errorcluster)  [unwired: 1 out]
        n425 = Cluster To Array(cluster=w802) -> (array=w801:i16[])
        n426 = To Unsigned Long Integer(number=w801) -> (unsigned 32bit integer=w782:u32[])
        n427 = local read "Scan steps (AOD)"() -> (w803:u64)
        n428 = Multiply(x=w793, y="N Acq Sets (Traps + Fl.)") -> (x*y=w791:u32)
        n429 = Divide(x=40000000.0, y=w793) -> (x/y=w785:dbl)
        "AI rate (Hz)" <- w785
        "Ave. Rate (Hz)" <- w785
        n430 = Add Array Elements(numeric array=w782) -> (sum=w794:u32)
        "Trap Sets" <- w794
        n431 = Reciprocal(x=w785) -> (1/x=→"Ave. Period (s)":dbl)
        n432 = property on="Scan steps (AOD)" class="DigNum (strict)"("Val(Sgnl)"=w803) -> ()  [unwired: 2 in, 2 out]
        n433 = Divide(x=w785, y="N Acq Sets (Traps + Fl.)") -> (x/y=w807:dbl)
        "Data Rate (Hz)" <- w807
        n434 = Reciprocal(x=w807) -> (1/x=→"Data Period (s)":dbl)
        n435 = local read "Save ave N"() -> (w806:dbl)
        n436 = Divide(x=w807, y=w806) -> (x/y=w805:dbl)
        "Save Data Rate (Hz)" <- w805
        n437 = Reciprocal(x=w805) -> (1/x=→"Save Data Period (s)":dbl)
        n438 = Multiply(x=w791, y="# Samples/trap") -> (x*y=w789:u32)
        "Counts/DMA" <- w789
        n439 = property on="Trap Disp. Downsample" class="DigNum (strict)"("Maximum"="# Samples/trap") -> ()  [unwired: 2 in, 2 out]
        n440 = Multiply(x=w794, y="# Samples/trap") -> (x*y=w783:u32)
        "# Samples/channel" <- w783
        n441 = Multiply(x=w783, y=u32 8) -> (x*y=→"Trap AI Elements/DMA read":u32)
        n442 = local read "APD Int. Count"() -> (w790:u32)
        n443 = Multiply(x=w783, y=u32 3) -> (x*y=→"Trap Pos Elements/DMA read":u32)
        n444 = Divide(x=w789, y=w790) -> (x/y=w780:dbl)
        "APD Samples/FIFO Acq." <- w780
        n445 = Divide(x=w789, y=40000000.0) -> (x/y=w787:dbl)
        "DMA Update Period (s)" <- w787
        n446 = Multiply(x=2.0, y=w780) -> (x*y=→"APD Elements/DMA read":dbl)
        n447 = property on="APD Disp. Downsample" class="DigNum (strict)"("Maximum"=w780) -> ()  [unwired: 2 in, 2 out]
        n448 = local read "N sets to save"() -> (w799:u32)
        n449 = Multiply(x=w787, y=w799) -> (x*y=→"Total Time (s)":dbl)
        "FPGA Averaging" <- FALSE ("FPGA Averaging")
      }
      event "Rescale on Mean": Value Change {
        n450 = event-data() -> ()  [unwired: 7 out]
        n451 = And(x=FALSE, y="Rescale on Mean") -> (x .and. y?=w814:bool)
        n452 = local write "Rescale on Mean"(w814) -> ()
        n453 = local read "Bead Mean (nm)"() -> (w819:dbl)
        n454 = Add(x="Amplitude (nm)", y=w819) -> (x+y=w817:dbl)
        n455 = Subtract(x=w819, y="Amplitude (nm)") -> (x-y=w816:dbl)
        n456 = property on="Bead Separation" class="WFChart (strict)"("YScale.Minimum"=w816) -> ()  [unwired: 2 in, 2 out]
        n457 = property on="Bead Separation" class="WFChart (strict)"("YScale.Maximum"=w817) -> ()  [unwired: 2 in, 2 out]
      }
      event "Detector Type": Value Change {
        n458 = event-data() -> ()  [unwired: 7 out]
        n459 = local read "AI labels"() -> (w820:string[])
        n460 = property on="High Res. Display" class="Ring (strict)"("Strings []"=w820) -> ()  [unwired: 2 in, 2 out]
        n461 = Build Array (concatenate)(w820, "none") -> (w821:string[])
        n462 = property on="FFT 1 Choice 1" class="Ring (strict)"("Strings []"=w821) -> ()  [unwired: 2 in, 2 out]
        n463 = property on="FFT 1 Choice 2" class="Ring (strict)"("Strings []"=w821) -> ()  [unwired: 2 in, 2 out]
        n464 = property on="FFT 2 Choice 1" class="Ring (strict)"("Strings []"=w821) -> ()  [unwired: 2 in, 2 out]
        n465 = property on="FFT 2 Choice 2" class="Ring (strict)"("Strings []"=w821) -> ()  [unwired: 2 in, 2 out]
        n466 = Bundle("APD 1", "APD 2") -> (w824:cluster{string, string})  [unwired: 1 out]
        n467 = Cluster To Array(cluster=w824) -> (array=w822:string[])
        n468 = Build Array (concatenate)(w822, w821) -> (w826:string[])
        n469 = Array Size(array=w826) -> (size(s)=w827:i32)
        n470 = property on="Signals to Plot" class="LstBox (strict)"("Item Names"=w826) -> ()  [unwired: 2 in, 2 out]
        n471 = property on="Signals to Plot" class="LstBox (strict)"("Number of Rows"=w827) -> ()  [unwired: 2 in, 2 out]
        n472 = property on="All Signals" class="WFChart (strict)"("LegNumRows"=w827) -> ()  [unwired: 2 in, 2 out]
      }
      event "Adjust Scale\nto Mean": Value Change {
        n473 = event-data() -> ()  [unwired: 7 out]
        n474 = local read "APD 1 Rate (Hz)"() -> (w836:dbl)
        n475 = Multiply(x=1000.0, y="Above (kHz)") -> (x*y=w834:dbl)
        n476 = Multiply(x=1000.0, y="Below (kHz)") -> (x*y=w832:dbl)
        n477 = Add(x=w834, y=w836) -> (x+y=w829:dbl)
        n478 = Subtract(x=w836, y=w832) -> (x-y=w830:dbl)
        n479 = property on="APD Chart" class="WFChart (strict)"("YScale.Minimum"=w830) -> ()  [unwired: 2 in, 2 out]
        n480 = property on="APD Chart" class="WFChart (strict)"("YScale.Maximum"=w829) -> ()  [unwired: 2 in, 2 out]
      }
